vi "filter.vi"(10 "IP":u32) -> ()   [LabVIEW 2022 SP3]
uses:
  nilvaiu.dll
panel:
  out "GetFilterPref":string[](array[string])
  in  "No selected devices message":string="No Selected Devices.\nYou must select at least one device."
  in  "Show all devices message":string="No Configured Devices.\nChanging filter option to Show Attributes For All Devices"
  out "output param 2":u32
  in  "Filter Options":u32(slide)=2 scale=0.0..2.0
  out "Item Symbols":i32[](array[numeric])
  out "Value":i32
  in  "CANCEL":bool
  in  "OK":bool
  in  "Listbox":i32(listbox)=1
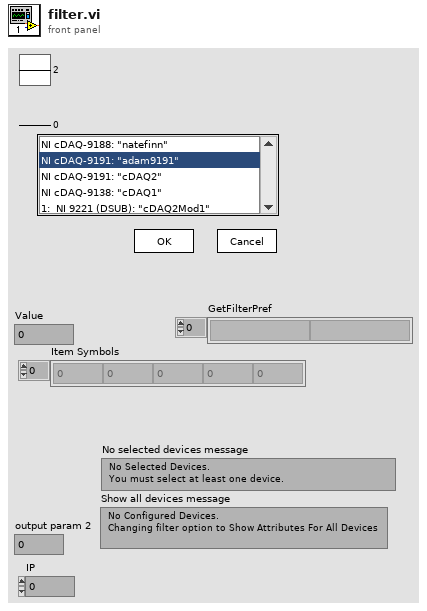
[diagram p1: front panel]
types:
  T1 = typedef "LVPoint32TypeDef.ctl" = cluster{"Horizontal":i32, "Vertical":i32}
  T2 = typedef "LVBoundsTypeDef.ctl" = cluster{"Width":u32, "Height":u32}
  T3 = typedef "LVPositionTypeDef.ctl" = cluster{"Left":i32, "Top":i32}
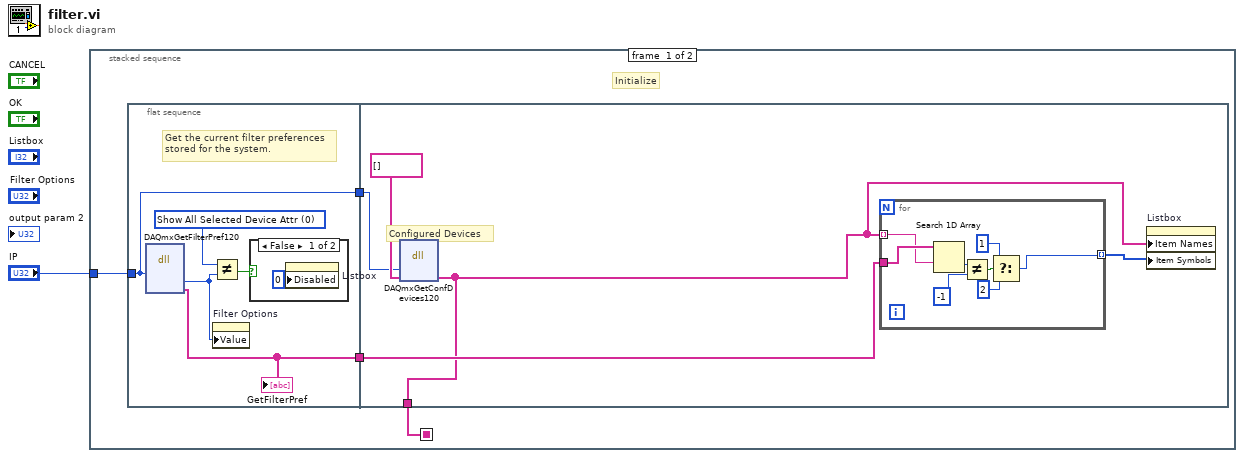
[diagram p0: block diagram]
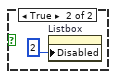
[diagram p2: hidden frame]
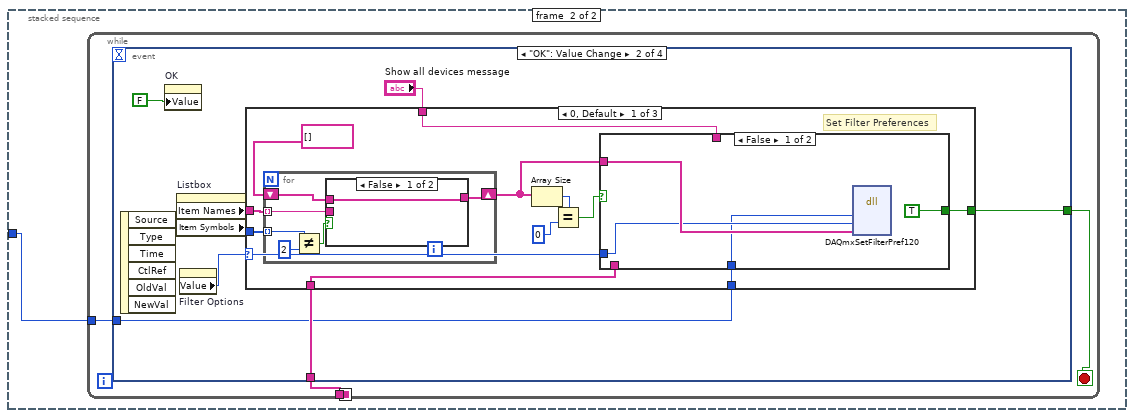
[diagram p3: hidden frame]
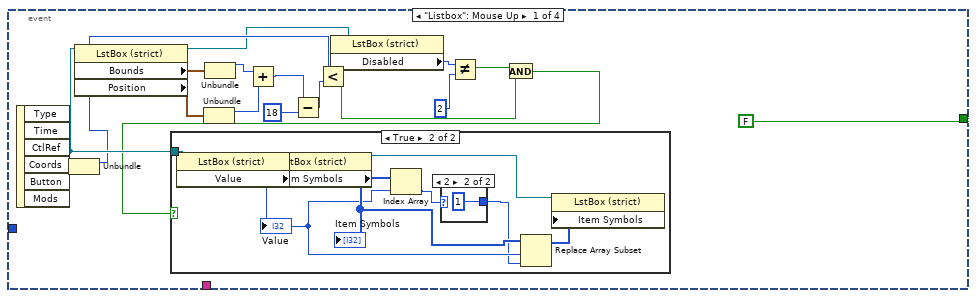
[diagram p4: hidden frame]
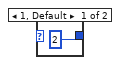
[diagram p6: hidden frame]
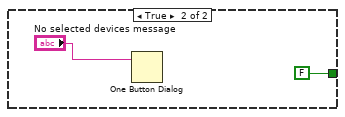
[diagram p7: hidden frame]
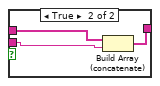
[diagram p8: hidden frame]
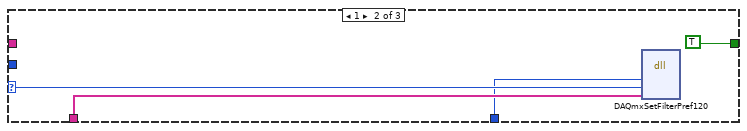
[diagram p9: hidden frame]
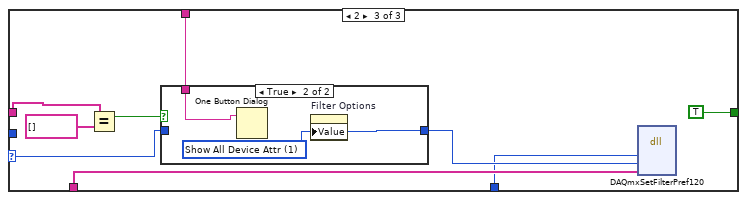
[diagram p10: hidden frame]
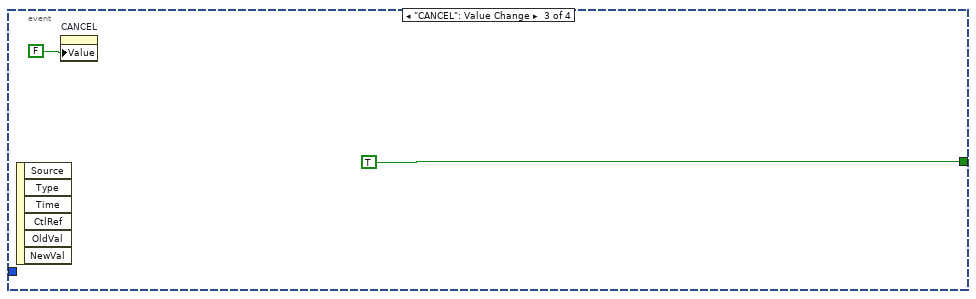
[diagram p12: hidden frame]
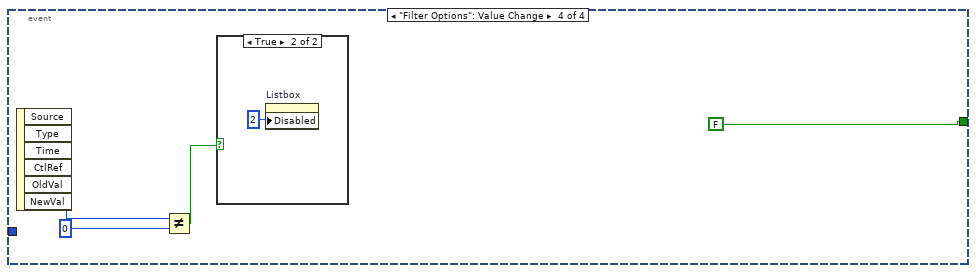
[diagram p13: hidden frame]
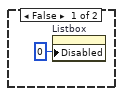
[diagram p14: hidden frame]
diagram:
  n1 = stacked-sequence {
    seq-local: [w4 _] -> [_ w27]
    tunnel: "IP" -> [w3 w26]
    frame #0 {
      # "Initialize"
      n2 = flat-sequence {
        tunnel: [w8] -> w5
        tunnel: w3 -> [w6]
        tunnel: [w6] -> w2
        tunnel: w5 -> [w17]
        tunnel: [w14] -> w4
        tunnel: w2 -> [w13]
        frame #0 {
          w9 = u16 0 items=["Show All Selected Device Attr", "Show All Device Attr", "Show Configured Device Attr"]
          # "Get the current filter preferences\nstored for the system."
          n3 = dll-call lib="nilvaiu.*" fn="DAQmxGetFilterPref120"("IP"=w6) -> ("option"=w7:i32, "GetFilterPref"=w8:string[])  [unwired: 4 in, 5 out]
          "GetFilterPref" <- w8
          n4 = Not Equal?(x=w9, y=w7) -> (x != y?=w10:bool)
          n5 = property on="Filter Options" class="Slide (strict)"("Value"=w7) -> ()  [unwired: 2 in, 2 out]
          n6 = case shown="False" w10 {
            frame False {
              n7 = property on="Listbox" class="LstBox (strict)"("Disabled"=u8 0) -> ()  [unwired: 2 in, 2 out]
            }
            frame True {
              n8 = property on="Listbox" class="LstBox (strict)"("Disabled"=2) -> ()  [unwired: 2 in, 2 out]
            }
          }
        }
        frame #1 {
          # "Configured Devices"
          n9 = dll-call lib="nilvaiu.*" fn="DAQmxGetConfDevices120"("IP"=w13, string[] []) -> (w14:string[])  [unwired: 4 in, 3 out]
          n10 = for {
            tunnel: [w25] -> w16 mode=indexing
            tunnel: w17 -> [w19]
            tunnel: w14 -> [w18] mode=indexing
            n11 = Search 1D Array(1D array=w19, element=w18) -> (index of element=w24:i32)  [unwired: 1 out]
            n12 = Not Equal?(x=w24, y=-1) -> (x != y?=w22:bool)
            n13 = Select(t=u32 1, s=w22, f=u32 2 ("y")) -> (s? t:f=w25:u32)
          }
          n14 = property on="Listbox" class="LstBox (strict)"("Item Names"=w14, "Item Symbols"=w16) -> ()  [unwired: 2 in, 2 out]
        }
      }
    }
    frame #1 {
      n15 = while {
        tunnel: w27 -> [w29]
        tunnel: w26 -> [w28]
        stop <- w30 stop-if-true
        n16 = event shown="[1] \"OK\": Value Change" {
          selector: _ -> [_ _ _ _]
          dyn-events: _ -> [_ _ _ _]
          timeout: _ -> [_ _ _ _]
          tunnel: [FALSE ("CANCEL") w61 TRUE ("CANCEL") FALSE ("CANCEL")] -> w30
          tunnel: w29 -> [_ w63 _ _]
          tunnel: w28 -> [_ w59 _ _]
          event "Listbox": Mouse Up {
            n17 = event-data() -> ("CtlRef"=w38:refnum<vi>, "Coords"=w41:T1)  [unwired: 5 out]
            n18 = Unbundle(w41) -> ("Horizontal"=w37:i32)  [unwired: 1 out]
            n19 = property class="LstBox (strict)"(reference=w38) -> (reference out=w34:refnum<vi>, "Bounds"=w47:T2, "Position"=w46:T3)  [unwired: 1 in, 1 out]
            n20 = Unbundle(w46) -> ("Left"=w44:i32)  [unwired: 1 out]
            n21 = Unbundle(w47) -> ("Width"=w45:u32)  [unwired: 1 out]
            n22 = Add(x=w45, y=w44) -> (x+y=w43:u32)
            n23 = Subtract(x=w43, y=u32 18) -> (x-y=w40:u32)
            n24 = Less?(x=w37, y=w40) -> (x < y?=w32:bool)
            n25 = property class="LstBox (strict)"(reference=w34) -> ("Disabled"=w35:u8)  [unwired: 1 in, 2 out]
            n26 = Not Equal?(x=w35, y=2) -> (x != y?=w33:bool)
            n27 = And(x=w33, y=w32) -> (x .and. y?=w31:bool)
            n28 = case shown="True" w31 {
              tunnel: w38 -> [_ w48]
              frame False {
              }
              frame True {
                n29 = property class="LstBox (strict)"(reference=w48) -> (reference out=w56:refnum<vi>, error out=w55:errorcluster, "Value"=w52:i32)  [unwired: 1 in]
                "Value" <- w52
                n30 = property class="LstBox (strict)"(reference=w56, error in=w55) -> (reference out=w49:refnum<vi>, "Item Symbols"=w53:i32[])  [unwired: 1 out]
                "Item Symbols" <- w53
                n31 = Index Array(array=w53, index=w52) -> (element=w54:i32)
                n32 = case shown="2" w54 {
                  tunnel: [2 1] -> w51
                  frame 1, Default {
                  }
                  frame 2 {
                  }
                }
                n33 = Replace Array Subset(array=w53, new element=w51, index=w52) -> (w50:i32[])
                n34 = property class="LstBox (strict)"(reference=w49, "Item Symbols"=w50) -> ()  [unwired: 1 in, 2 out]
              }
            }
          }
          event "OK": Value Change {
            n35 = event-data() -> ()  [unwired: 7 out]
            n36 = property on="OK" class="Bool (strict)"("Value"=FALSE ("OK")) -> ()  [unwired: 2 in, 2 out]
            n37 = property on="Listbox" class="LstBox (strict)"() -> ("Item Names"=w64:string[], "Item Symbols"=w65:i32[])  [unwired: 2 in, 2 out]
            n38 = property on="Filter Options" class="Slide (strict)"() -> ("Value"=w66:u32)  [unwired: 2 in, 2 out]
            n39 = case shown="0, Default" w66 {
              selector: w66 -> [w77 w96 w105]
              tunnel: w65 -> [w78 _ _]
              tunnel: w64 -> [w71 _ w104]
              tunnel: w63 -> [w70 w97 w101]
              tunnel: "Show all devices message" -> [w72 _ w103]
              tunnel: [w68 TRUE ("CANCEL") TRUE ("CANCEL")] -> w61
              tunnel: w59 -> [w67 w95 w99]
              frame 0, Default {
                # "Set Filter Preferences"
                n40 = for {
                  tunnel: w71 -> [w89] mode=indexing
                  shift-right: [w85] -> w69
                  shift-left: string[] [] -> [w90]
                  tunnel: w78 -> [w88] mode=indexing
                  n41 = Not Equal?(x=w88, y=2) -> (x != y?=w86:bool)
                  n42 = case shown="False" w86 {
                    tunnel: w90 -> [w91 w94]
                    tunnel: w89 -> [_ w93]
                    tunnel: [w91 w92] -> w85
                    frame False {
                    }
                    frame True {
                      n43 = Build Array (concatenate)(w94, w93) -> (w92:string[])
                    }
                  }
                }
                n44 = Array Size(array=w69) -> (size(s)=w75:i32)
                n45 = Equal?(x=w75, y=0) -> (x = y?=w73:bool)
                n46 = case shown="False" w73 {
                  tunnel: w77 -> [w80 _]
                  tunnel: w72 -> [_ _]
                  tunnel: w70 -> [_ _]
                  tunnel: w69 -> [w81 _]
                  tunnel: [TRUE ("CANCEL") FALSE ("CANCEL")] -> w68
                  tunnel: w67 -> [w79 _]
                  frame False {
                    n47 = dll-call lib="nilvaiu.*" fn="DAQmxSetFilterPref120"("IP"=w79, "option"=w80, w81) -> ()  [unwired: 6 in, 3 out]
                  }
                  frame True {
                    n48 = One Button Dialog(message="No selected devices message") -> ()  [unwired: 2 out]
                  }
                }
              }
              frame 1 {
                n49 = dll-call lib="nilvaiu.*" fn="DAQmxSetFilterPref120"("IP"=w95, "option"=w96, w97) -> ()  [unwired: 6 in, 3 out]
              }
              frame 2 {
                n50 = Equal?(x=w104, y=string[] []) -> (x = y?=w106:bool)
                n51 = case shown="True" w106 {
                  tunnel: [w108 w110] -> w100
                  tunnel: w105 -> [w108 _]
                  tunnel: w103 -> [_ w109]
                  frame False {
                  }
                  frame True {
                    w110 = 1 items=["Show All Selected Device Attr", "Show All Device Attr", "Show Configured Device Attr"]
                    n52 = One Button Dialog(message=w109) -> ()  [unwired: 2 out]
                    n53 = property on="Filter Options" class="Slide (strict)"("Value"=w110) -> ()  [unwired: 2 in, 2 out]
                  }
                }
                n54 = dll-call lib="nilvaiu.*" fn="DAQmxSetFilterPref120"("IP"=w99, "option"=w100, w101) -> ()  [unwired: 6 in, 3 out]
              }
            }
          }
          event "CANCEL": Value Change {
            n55 = event-data() -> ()  [unwired: 7 out]
            n56 = property on="CANCEL" class="Bool (strict)"("Value"=FALSE ("CANCEL")) -> ()  [unwired: 2 in, 2 out]
          }
          event "Filter Options": Value Change {
            n57 = event-data() -> ("NewVal"=w115:u32)  [unwired: 6 out]
            n58 = Not Equal?(x=w115, y=u32 0) -> (x != y?=w113:bool)
            n59 = case shown="True" w113 {
              frame False {
                n60 = property on="Listbox" class="LstBox (strict)"("Disabled"=u8 0) -> ()  [unwired: 2 in, 2 out]
              }
              frame True {
                n61 = property on="Listbox" class="LstBox (strict)"("Disabled"=u8 2) -> ()  [unwired: 2 in, 2 out]
              }
            }
          }
        }
      }
    }
  }
